vi "appendCircArr.vi"   [LabVIEW 2016, in "OfcFunc.lvlib" / "MatOper.lvclass"]
uses:
  MatOper.lvclass
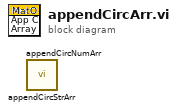
[diagram p0: block diagram]
diagram:
  n1 = call "appendCircStrArr.vi"() -> ()  [unwired: 9 in, 3 out]
  n2 = call "appendCircNumArr.vi"() -> ()  [unwired: 9 in, 3 out]
